vi "To Pretty String (Array).vi"(0 "Variant in":variant, 5 "indent":i32, 7 "enable LabVIEW extensions? (T)":bool=TRUE, 9 "pretty print? (T)":bool=TRUE, 11 "error in (no error)":errorcluster) -> (4 "Pretty Print String":string, 15 "error out":errorcluster)   [LabVIEW 2020, in "Variant JSON API.lvlib"]
doc: "Pretty prints the given JSON data in an easier to read format."
uses:
  Variant JSON API.lvlib
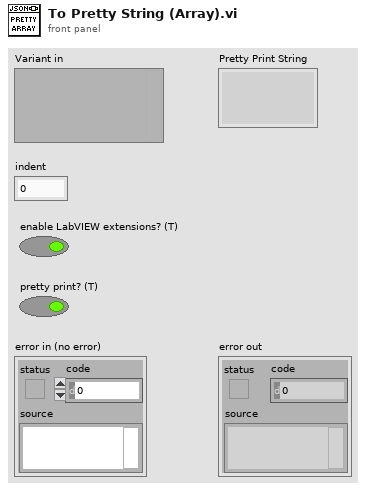
[diagram p1: front panel]
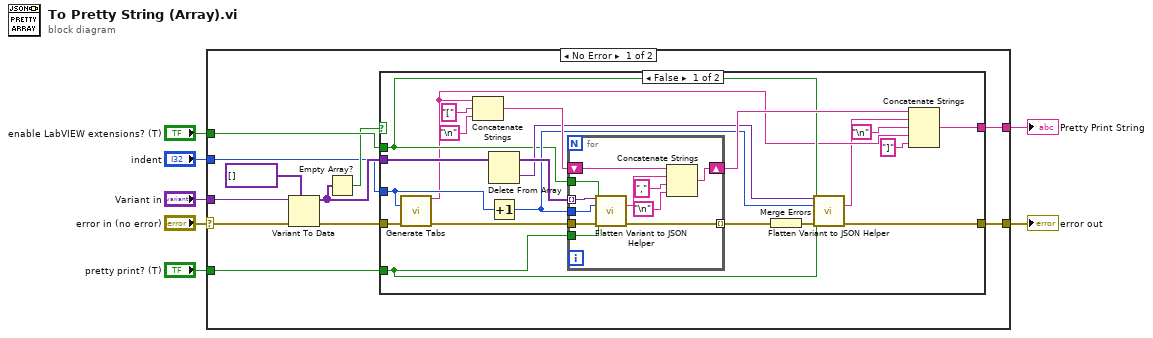
[diagram p0: block diagram]
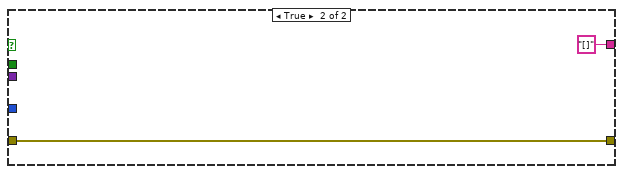
[diagram p2: hidden frame]
diagram:
  n1 = case shown="No Error" "error in (no error)" {
    selector: "error in (no error)" -> [w14 w53]
    tunnel: [w18 _] -> w7
    tunnel: [w17 w53] -> w6
    tunnel: "enable LabVIEW extensions? (T)" -> [w16 _]
    tunnel: "Variant in" -> [w15 _]
    tunnel: "indent" -> [w10 _]
    tunnel: "pretty print? (T)" -> [w9 _]
    frame No Error {
      n2 = Variant To Data(error in=w14, type=variant[] [], Variant=w15) -> (data=w11:variant[], error out=w13:errorcluster)
      n3 = Empty Array?(array=w11) -> (empty?=w12:bool)
      n4 = case shown="False" w12 {
        tunnel: [w39 "[]"] -> w18
        tunnel: [w24 w51] -> w17
        tunnel: w11 -> [w29 _]
        tunnel: w16 -> [w22 _]
        tunnel: w13 -> [w38 w51]
        tunnel: w10 -> [w37 _]
        tunnel: w9 -> [w23 _]
        frame False {
          n5 = call "Generate Tabs.vi"("indent"=w37, "error in (no error)"=w38) -> ("Tabs"=w20:string, "error out"=w35:errorcluster)  [unwired: 12 in]
          n6 = Concatenate Strings(w20, "[" ("string"), "\n") -> (w33:string)
          n7 = Delete From Array(array=w29) -> (deleted portion=w27:variant, array with subset deleted=w28:variant[])  [unwired: 2 in]
          n8 = Increment(x=w37) -> (x+1=w26:i32)
          n9 = for {
            tunnel: w28 -> [w50] mode=indexing
            tunnel: w26 -> [w49]
            tunnel: w35 -> [w48]
            shift-right: [w47] -> w32
            shift-left: w33 -> [w46]
            tunnel: [w45] -> w31 mode=indexing
            tunnel: w23 -> [w44]
            tunnel: w22 -> [w43]
            n10 = call "Flatten Variant to JSON Helper.vi"("Variant in"=w50, "indent"=w49, "enable LabVIEW extensions? (T)"=w43, "pretty print? (T)"=w44, "error in (no error)"=w48) -> ("String"=w40:string, "error out"=w45:errorcluster)  [unwired: 8 in, 1 out]
            n11 = Concatenate Strings(w46, w40, "," ("string"), "\n") -> (w47:string)
          }
          n12 = Merge Errors(w31) -> (w25:errorcluster)
          n13 = call "Flatten Variant to JSON Helper.vi"("Variant in"=w27, "indent"=w26, "enable LabVIEW extensions? (T)"=w22, "pretty print? (T)"=w23, "error in (no error)"=w25) -> ("String"=w19:string, "error out"=w24:errorcluster)  [unwired: 8 in, 1 out]
          n14 = Concatenate Strings(w32, w19, "\n", w20, "]" ("string")) -> (w39:string)
        }
        frame True {
        }
      }
    }
    frame Error {
    }
  }
  "error out" <- w6
  "Pretty Print String" <- w7
